vi "Get-Acquisition.vi"(8 "error in (no error)":errorcluster, 11 "UI ref. in":refnum<data-value>) -> (0 "error out":errorcluster, 1 "Acquisition":bool, 3 "UI ref.":refnum<data-value>)   [LabVIEW 2013, in "CameraVision.lvlib" / "CV-UI.lvclass"]
uses:
  CV-UI.lvclass
  CV-UI.lvclass/CV-UI.ctl
  Notifier-with-memory-boolean.vi
  Read Acquisition.vi
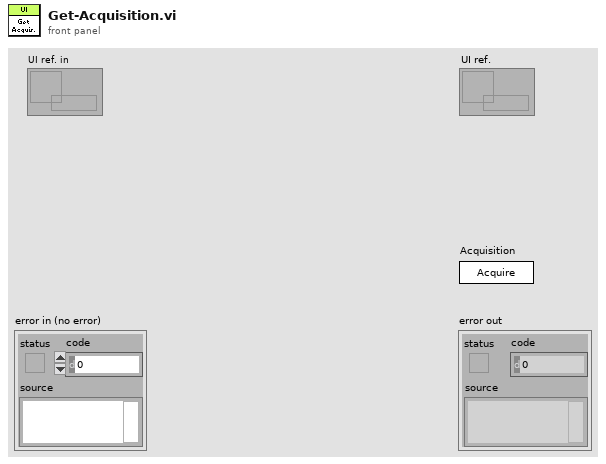
[diagram p1: front panel]
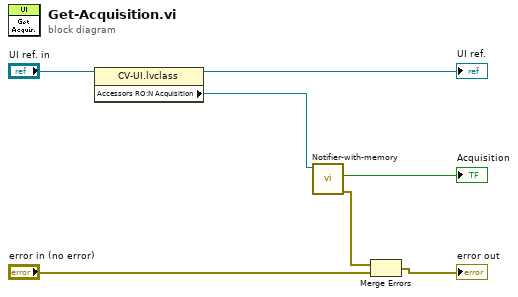
[diagram p0: block diagram]
diagram:
  n1 = property class="CV-UI.lvclass"(reference="UI ref. in") -> (reference out=→"UI ref.":refnum<data-value>, "Accessors RO:N Acquisition"=w3:refnum<notifier>)  [unwired: 1 in, 1 out]
  n2 = call-poly "Notifier-with-memory.vi"("Notifier in"=w3) -> ("error IO"=w7:errorcluster, "Notification"=→"Acquisition":bool)  [unwired: 9 in]
  n3 = Merge Errors(w7, "error in (no error)") -> (→"error out":errorcluster)
